vi "5 Pin Control.vi"() -> ()   [LabVIEW 2020]
panel:
  in  "Write Pin":bool[](array[boolean])=[TRUE]
  in  "Clear Pin":bool[](array[boolean])=[TRUE]
  in  "Sync Pin":bool[](array[boolean])=[TRUE]
  in  "Data Pin":bool[](array[boolean])=[TRUE]
  in  "stop":bool
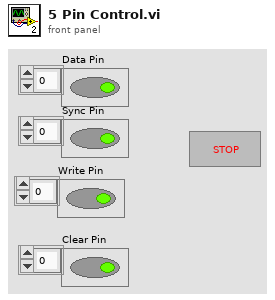
[diagram p1: front panel]
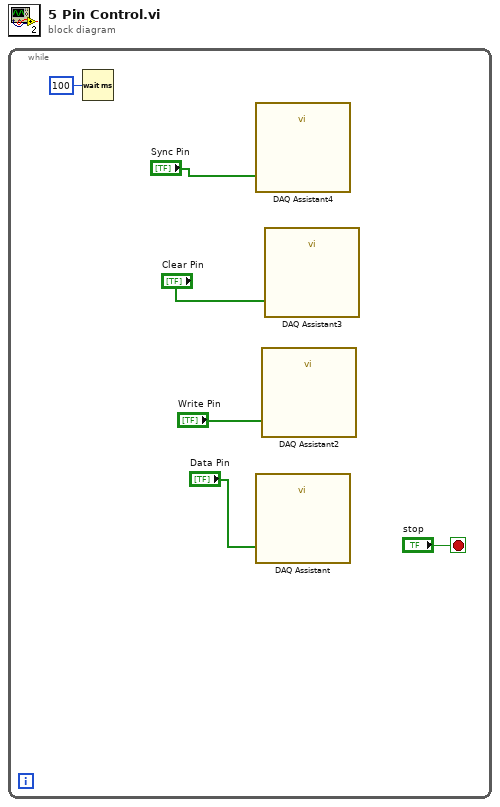
[diagram p0: block diagram]
diagram:
  n1 = while {
    stop <- "stop" stop-if-true
    n2 = Wait (ms)(milliseconds to wait=u32 100) -> ()  [unwired: 1 out]
    n3 = call "DAQ Assistant4"("data"="Sync Pin") -> ()  [unwired: 17 in, 2 out]
    n4 = call "DAQ Assistant"("data"="Data Pin") -> ()  [unwired: 17 in, 2 out]
    n5 = call "DAQ Assistant2"("data"="Write Pin") -> ()  [unwired: 17 in, 2 out]
    n6 = call "DAQ Assistant3"("data"="Clear Pin") -> ()  [unwired: 17 in, 2 out]
  }
